vi "setData.vi"(9 "COM":bool, 10 "VISA name":refnum<visa-resource-name>, 11 "Array":string[](array[string])) -> (3 "return":i32)   [LabVIEW 2016]
panel:
  out "return 2":i32
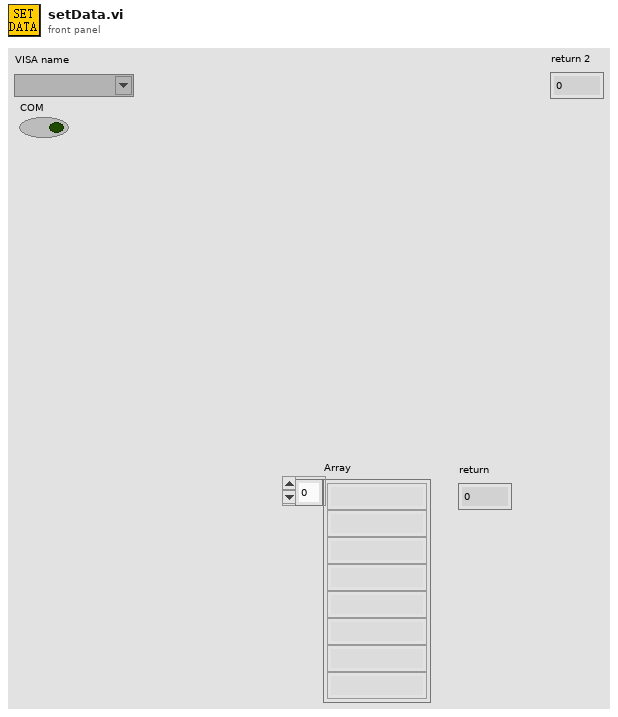
[diagram p1: front panel]
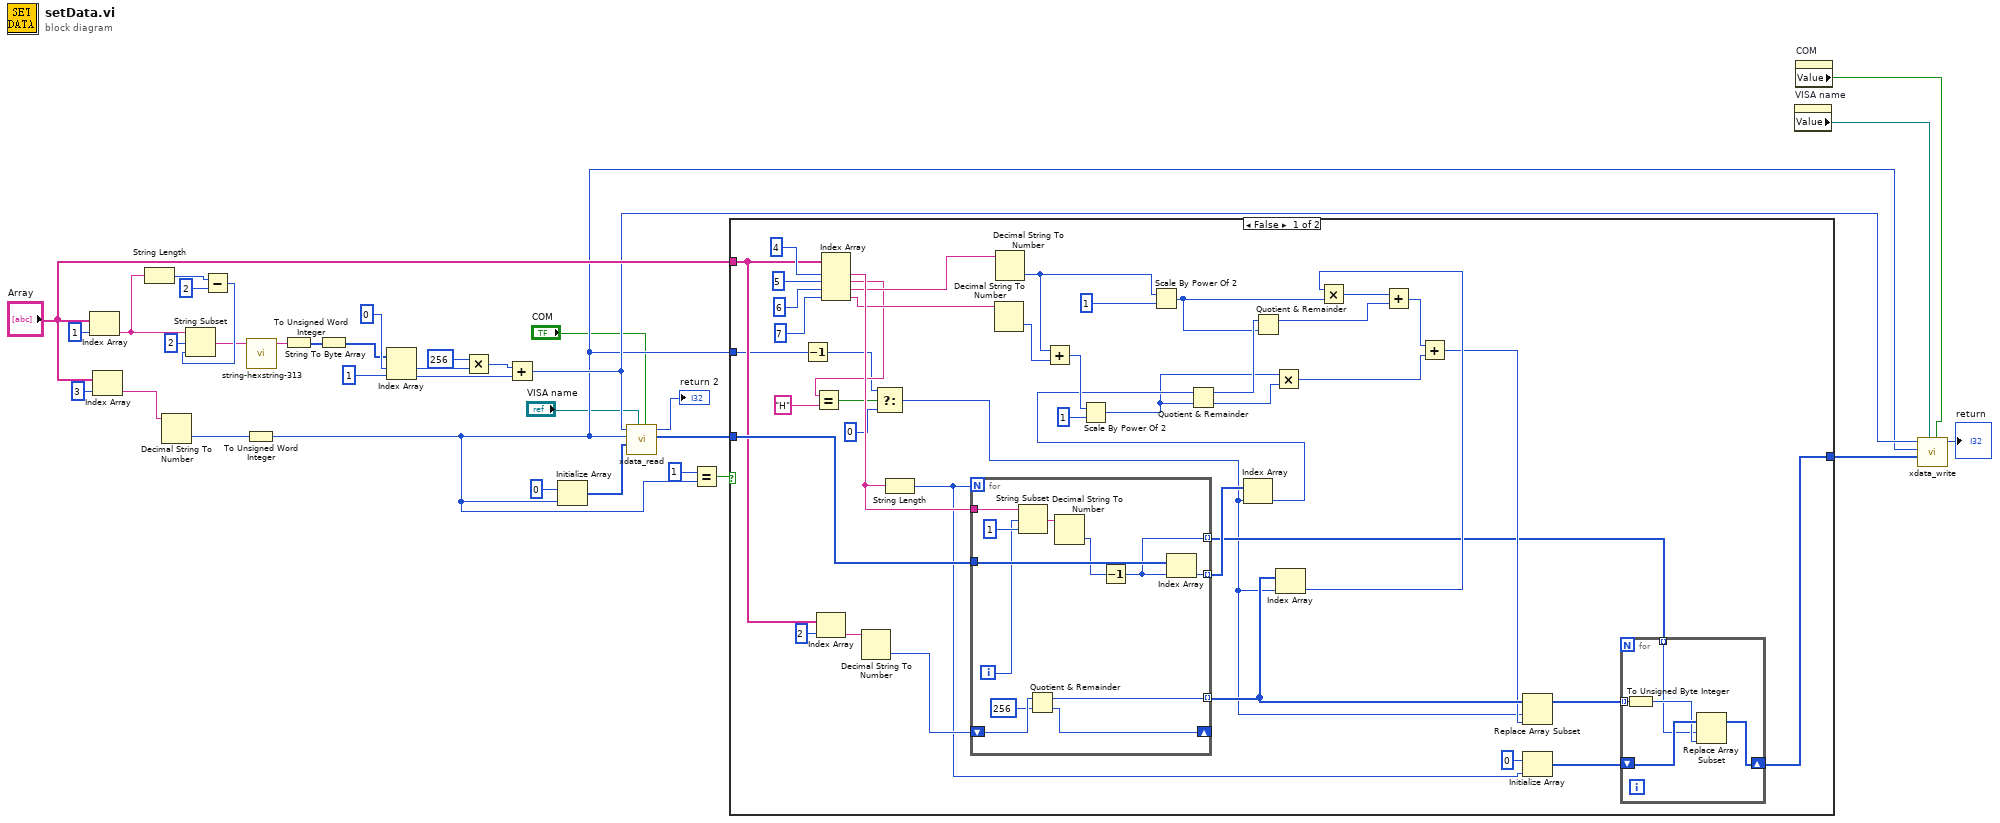
[diagram p0: block diagram]
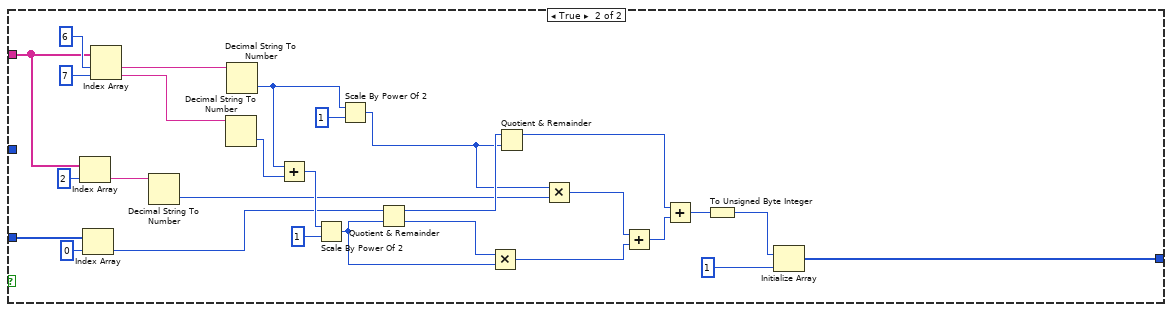
[diagram p2: hidden frame]
diagram:
  n1 = Index Array(array="Array", index=1) -> (element=w33:string)
  n2 = Index Array(array="Array", index=3) -> (element=w17:string)
  n3 = String Length(string=w33) -> (length=w32:i32)
  n4 = Decimal String To Number(string=w17) -> (number=w16:i32)  [unwired: 2 in, 1 out]
  n5 = Subtract(x=w32, y=2) -> (x-y=w30:i32)
  n6 = String Subset(string=w33, offset (0)=2, length (rest)=w30) -> (substring=w28:string)
  n7 = To Unsigned Word Integer(number=w16) -> (unsigned 16bit integer=w6:u16)
  n8 = call "string-hexstring-313.vi"("字符串"=w28) -> ("十六进制整型字符串"=w27:string)  [unwired: 10 in]
  n9 = String To Byte Array(string=w27) -> (unsigned byte array=w26:u8[])
  n10 = To Unsigned Word Integer(number=w26) -> (unsigned 16bit integer=w23:u16[])
  n11 = Index Array(array=w23, index #1=0 ("index"), index #2=1 ("index")) -> (element #1=w22:u16, element #2=w19:u16)
  n12 = Multiply(x=u16 256, y=w22) -> (x*y=w20:u16)
  n13 = Add(x=w20, y=w19) -> (x+y=w8:u16)
  n14 = Initialize Array(u8 0 ("element"), w6) -> (w14:u8[])
  n15 = call "xdata_read.vi"("COM"="COM", "VISA name"="VISA name", "data"=w14, "wLen"=w6, "wAddr"=w8) -> ("data out"=w11:u8[], "return"=→"return 2":i32)  [unwired: 5 in]
  n16 = Equal?(x=u16 1, y=w6) -> (x = y?=w13:bool)
  n17 = case shown="False" w13 {
    tunnel: w11 -> [w64 w122]
    tunnel: "Array" -> [w55 w109]
    tunnel: [w42 w96] -> w9
    tunnel: w6 -> [w38 _]
    frame False {
      n18 = Decrement(x=w38) -> (x-1=w37:u16)
      n19 = Index Array(array=w55, index=2) -> (element=w57:string)
      n20 = Index Array(array=w55, index #1=4 ("index"), index #2=5 ("index"), index #3=6 ("index"), index #4=7 ("index")) -> (element #1=w67:string, element #2=w41:string, element #3=w66:string, element #4=w65:string)
      n21 = Equal?(x=w41, y="H") -> (x = y?=w39:bool)
      n22 = Decimal String To Number(string=w57) -> (number=w54:i32)  [unwired: 2 in, 1 out]
      n23 = Select(t=w37, s=w39, f=u16 0) -> (s? t:f=w35:u16)
      n24 = String Length(string=w67) -> (length=w46:i32)
      n25 = for {
        N: w46 -> [_]
        tunnel: w67 -> [w94]
        tunnel: [w90] -> w62 mode=indexing
        tunnel: w64 -> [w91]
        tunnel: [w86] -> w49 mode=indexing
        shift-right: [w85] -> _
        shift-left: w54 -> [w88]
        tunnel: [w83] -> w44 mode=indexing
        i -> [w89]
        n26 = String Subset(string=w94, offset (0)=w89, length (rest)=1 ("length (rest)")) -> (substring=w92:string)
        n27 = Quotient & Remainder(x=w88, y=256) -> (x-y*floor(x/y)=w86:i32, floor(x/y)=w85:i32)
        n28 = Decimal String To Number(string=w92) -> (number=w84:i32)  [unwired: 2 in, 1 out]
        n29 = Decrement(x=w84) -> (x-1=w83:i32)
        n30 = Index Array(array=w91, index=w83) -> (element=w90:u8)
      }
      n31 = Decimal String To Number(string=w65) -> (number=w72:i32)  [unwired: 2 in, 1 out]
      n32 = Decimal String To Number(string=w66) -> (number=w73:i32)  [unwired: 2 in, 1 out]
      n33 = Add(x=w73, y=w72) -> (x+y=w71:i32)
      n34 = Scale By Power Of 2(n=w71, x=u16 1) -> (x*2^n=w60:u16)
      n35 = Scale By Power Of 2(n=w73, x=u8 1) -> (x*2^n=w59:u8)
      n36 = Index Array(array=w62, index=w35) -> (element=w63:u8)
      n37 = Quotient & Remainder(x=w63, y=w60) -> (x-y*floor(x/y)=w70:u16, floor(x/y)=w61:u16)
      n38 = Quotient & Remainder(x=w70, y=w59) -> (x-y*floor(x/y)=w51:u16)  [unwired: 1 out]
      n39 = Multiply(x=w60, y=w61) -> (x*y=w58:u16)
      n40 = Index Array(array=w49, index=w35) -> (element=w53:i32)
      n41 = Multiply(x=w53, y=w59) -> (x*y=w52:i32)
      n42 = Add(x=w52, y=w51) -> (x+y=w50:i32)
      n43 = Add(x=w50, y=w58) -> (x+y=w48:i32)
      n44 = Replace Array Subset(array=w49, new element=w48, index=w35) -> (w45:i32[])
      n45 = Initialize Array(u8 0 ("element"), w46) -> (w43:u8[])
      n46 = for {
        tunnel: w45 -> [w81] mode=indexing
        tunnel: w44 -> [w79] mode=indexing
        shift-right: [w78] -> w42
        shift-left: w43 -> [w82]
        n47 = To Unsigned Byte Integer(number=w81) -> (unsigned 8bit integer=w80:u8)
        n48 = Replace Array Subset(array=w82, new element=w80, index=w79) -> (w78:u8[])
      }
    }
    frame True {
      n49 = Index Array(array=w109, index=2) -> (element=w107:string)
      n50 = Index Array(array=w122, index=0) -> (element=w111:u8)
      n51 = Index Array(array=w109, index #1=6 ("index"), index #2=7 ("index")) -> (element #1=w117:string, element #2=w118:string)
      n52 = Decimal String To Number(string=w107) -> (number=w103:i32)  [unwired: 2 in, 1 out]
      n53 = Decimal String To Number(string=w118) -> (number=w113:i32)  [unwired: 2 in, 1 out]
      n54 = Decimal String To Number(string=w117) -> (number=w114:i32)  [unwired: 2 in, 1 out]
      n55 = Add(x=w114, y=w113) -> (x+y=w112:i32)
      n56 = Scale By Power Of 2(n=w112, x=u16 1) -> (x*2^n=w105:u16)
      n57 = Scale By Power Of 2(n=w114, x=u8 1) -> (x*2^n=w104:u8)
      n58 = Quotient & Remainder(x=w111, y=w105) -> (x-y*floor(x/y)=w110:u16, floor(x/y)=w106:u16)
      n59 = Multiply(x=w106, y=w105) -> (x*y=w101:u16)
      n60 = Quotient & Remainder(x=w110, y=w104) -> (x-y*floor(x/y)=w99:u16)  [unwired: 1 out]
      n61 = Multiply(x=w104, y=w103) -> (x*y=w102:i32)
      n62 = Add(x=w102, y=w101) -> (x+y=w100:i32)
      n63 = Add(x=w99, y=w100) -> (x+y=w98:i32)
      n64 = To Unsigned Byte Integer(number=w98) -> (unsigned 8bit integer=w95:u8)
      n65 = Initialize Array(w95, 1 ("dimension size")) -> (w96:u8[])
    }
  }
  n66 = property on="VISA name" class="VISAName"() -> ("Value"=w2:refnum<visa-resource-name>)  [unwired: 2 in, 2 out]
  n67 = property on="COM" class="Bool (strict)"() -> ("Value"=w1:bool)  [unwired: 2 in, 2 out]
  n68 = call "xdata_write.vi"("COM"=w1, "VISA name"=w2, "data"=w9, "wLen"=w6, "wAddr"=w8) -> ("return"=→"return":i32)  [unwired: 6 in]
